vi "test_LoadCommandlineArgs_MixedParameterSize.vi"() -> (3 "Pass?":bool)   [LabVIEW 2019, in "Tests.SolutionBuilder.lvlib"]
uses:
  Tests.SolutionBuilder.lvlib
  SolutionBuilder/Community/Options.ctl
  SolutionBuilder/SolutionBuilder.lvclass
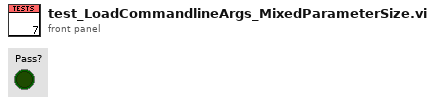
[diagram p1: front panel]
types:
  T1 = typedef "SolutionBuilder.lvlib/SolutionBuilder.lvclass/Options.ctl" = cluster{"Path":path, "Preview?":bool, "Quiet?":bool, "Log file":path, "Success file":path, "Rebuild?":bool, "Keep split projects?":bool}
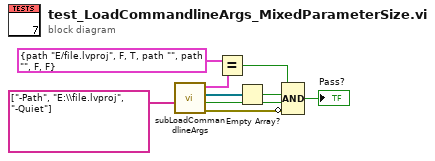
[diagram p0: block diagram]
diagram:
  n1 = call "subLoadCommandlineArgs.vi"("App.Args"=string[] ["-Path", "E:\\file.lvproj", "-Quiet"]) -> ("error out"=w1:errorcluster, "From command line?"=w7:bool, "Pre-built libraries"=w4:refnum<class "ProjectItem.lvclass">[], "Options"=w3:T1)  [unwired: 6 in, 1 out]
  n2 = Equal?(x=T1 {"Path"=path "E:/file.lvproj", "Preview?"=FALSE, "Quiet?"=TRUE, "Log file"=path "", "Success file"=path "", "Rebuild?"=FALSE, "Keep split projects?"=FALSE} ("Options"), y=w3) -> (x = y?=w6:bool)
  n3 = Empty Array?(array=w4) -> (empty?=w5:bool)
  n4 = Compound Arithmetic op=AND(w6, w5, w7, invert w1) -> (→"Pass?":bool)
